vi "disk_check.vi"() -> ()   [LabVIEW 2017]
uses:
  Globals/Global - All RT Loop Stop.vi
panel:
  out "error out":errorcluster
  out "Free Physical Memory or Largest Contiguous Memory (bytes)":i64(graph)
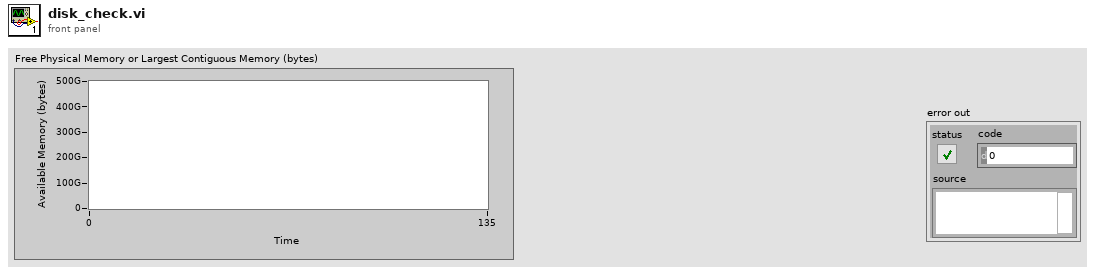
[diagram p1: front panel]
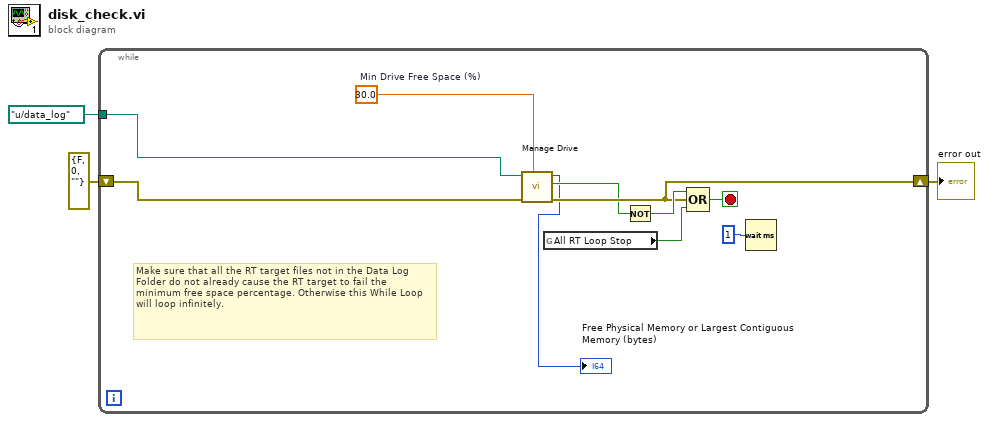
[diagram p0: block diagram]
diagram:
  n1 = while {
    shift-right: [w8] -> w1
    shift-left: errorcluster {"status"=FALSE, "code"=0, "source"=""} ("error out") -> [w9]
    tunnel: path "u:/data_log" ("AVI Path") -> [w6]
    stop <- w13 stop-if-true
    w7 = 30.0  # Min Drive Free Space (%)
    # "Make sure that all the RT target files not in the Data Log Folder do not already cause the RT target to fail the minimum free space percentage. Otherwise this While Loop will loop infinitely."
    n2 = call "Manage Drive.vi"("Min Drive Free Space (%)"=w7, "error in"=w9, "Data Folder"=w6) -> ("error out"=w8:errorcluster, "Drive Space Below Limit"=w5:bool, "size (bytes)"=→"Free Physical Memory or Largest Contiguous Memory (bytes)":i64)  [unwired: 6 in]
    n3 = global read "Global - All RT Loop Stop.vi" "All RT Loop Stop"() -> (w10:bool)
    n4 = Not(x=w5) -> (.not. x?=w12:bool)
    n5 = Compound Arithmetic op=OR(w12, w8, w10) -> (w13:bool)
    n6 = Wait (ms)(milliseconds to wait=u32 1) -> ()  [unwired: 1 out]
  }
  "error out" <- w1
